vi "XB PC Cmd.vi"(0 "VISA resource name":refnum<visa-resource-name>, 1 "Command String":string, 2 "error in (no error)":errorcluster) -> (3 "VISA resource name out":refnum<visa-resource-name>, 4 "String Received":string, 5 "Time out?":bool, 6 "error out":errorcluster)   [LabVIEW 2011]
doc: "This VI accepts a command string which ends with a \"^\" and sends to NXT via an XBee. After a fixed delay,\nit reads the return string which ends with a \">\". If too long a time elaspes, an error is generated."
panel:
  out "Send OK?":bool
  in  "Time":u32=200
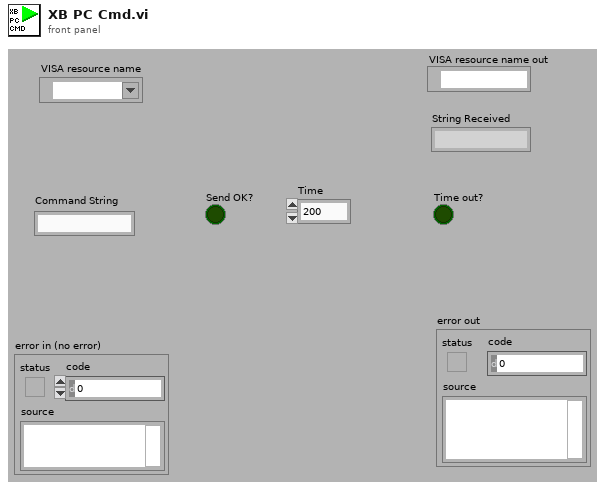
[diagram p1: front panel]
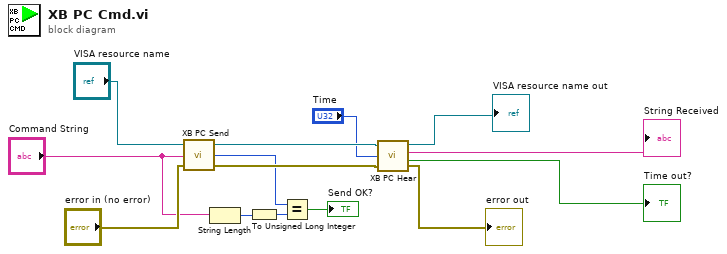
[diagram p0: block diagram]
diagram:
  n1 = call "XB PC Send.vi"("error in (no error)"="error in (no error)", "String"="Command String", "VISA resource name"="VISA resource name") -> ("error out"=w6:errorcluster, "return count"=w4:u32, "VISA resource name out"=w12:refnum<visa-resource-name>)
  n2 = String Length(string="Command String") -> (length=w2:i32)
  n3 = To Unsigned Long Integer(number=w2) -> (unsigned 32bit integer=w3:u32)
  n4 = Equal?(x=w4, y=w3) -> (x = y?=→"Send OK?":bool)
  n5 = call "XB PC Hear.vi"("VISA resource name"=w12, "Time"="Time", "error in (no error)"=w6) -> ("VISA resource name out"=→"VISA resource name out":refnum<visa-resource-name>, "String Received"=→"String Received":string, "Time out?"=→"Time out?":bool, "error out"=→"error out":errorcluster)
